vi "Set Busy Cursor.vi"(8 "error in (no error)":errorcluster, 11 "Busy":bool) -> (0 "error out":errorcluster)   [LabVIEW 2015, in "Main Controller Actor API.lvclass"]
uses:
  Main Controller Actor API.lvclass
  Re-use Libraries/Minimal Actor Framework/Messaging/Message/Message.lvclass/Message.ctl
  Globals.vi
  Re-use Libraries/Minimal Actor Framework/Messaging/Message/Message.lvclass
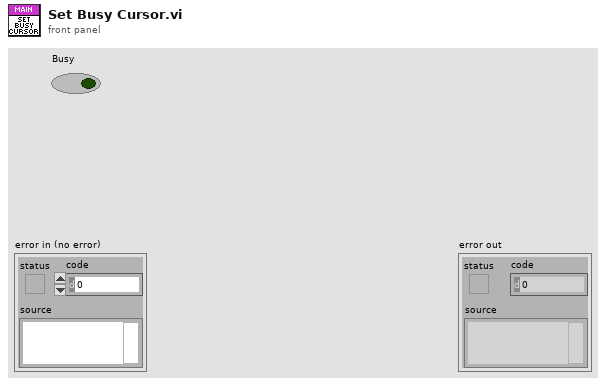
[diagram p1: front panel]
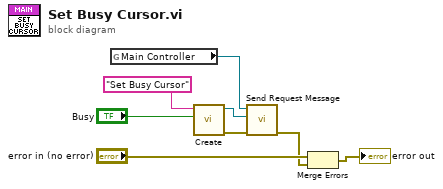
[diagram p0: block diagram]
diagram:
  n1 = global read "Globals.vi" "Main Controller"() -> (w6:refnum<class "Main Controller Actor API.lvclass">)
  n2 = call "Create.vi"("Data"="Busy", "Name"="Set Busy Cursor" ("Parameter")) -> ("error out"=w3:errorcluster, "Message out"=w7:refnum<class "Message.lvclass">)  [unwired: 8 in]
  n3 = call-dynamic "Send Request Message.vi"("error in (no error)"=w3, "Message"=w7, "Actor API in"=w6) -> ("error out"=w2:errorcluster)  [unwired: 8 in]
  n4 = Merge Errors("error in (no error)", w2) -> (→"error out":errorcluster)
